vi "FPGA Test.vi"() -> (1 "Resource":string, 2 "ProdName":string)   [LabVIEW 2017]
uses:
  <vilib>/nisyscfg/nisyscfg.lvlib
  <resource>/objmgr/niflexriosae.rc
  <resource>/objmgr/nicriosae.rc
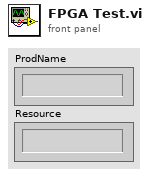
[diagram p1: front panel]
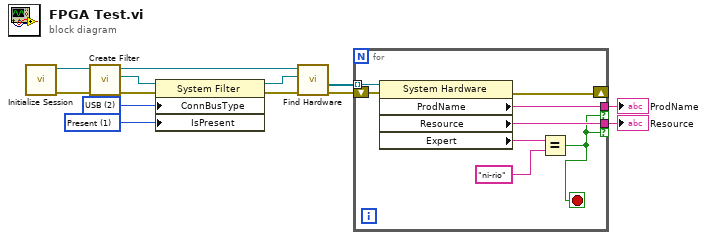
[diagram p0: block diagram]
diagram:
  w6 = 1 items=["Initializing"=-2, "Unknown"=-1, "Not Present"=0, "Present"=1] ("Devices & Chassis:Is Present")
  w7 = u32 2 items=["BuiltIn/System", "PXI/PCI", "USB", "GPIB", "VXI", "Serial", "TCP/IP", "cRIO", "SCXI", "cDAQ", "SwitchBlock", "SCC", "FireWire", "Accessory", "CAN", "SwitchBlock Device"] ("Devices & Chassis:Connects To Bus Type")
  n1 = call <vilib>:"Initialize Session.vi"() -> ("error out"=w5:errorcluster, "Session out"=w9:refnum<k21>)  [unwired: 10 in]
  n2 = call <vilib>:"Create Filter.vi"("error in (no error)"=w5, "Session in"=w9) -> ("error out"=w13:errorcluster, "Filter out"=w12:refnum<k20>, "Session out"=w8:refnum<k21>)  [unwired: 7 in]
  n3 = property class="System Filter"(reference=w12, error in=w13, "ConnBusType"=w7, "IsPresent"=w6) -> (reference out=w11:refnum<k20>, error out=w4:errorcluster)
  n4 = call <vilib>:"Find Hardware.vi"("error in (no error)"=w4, "Filter in"=w11, "Session in"=w8) -> ("error out"=w3:errorcluster, "Resources out"=w10:refnum<k20>[])  [unwired: 5 in, 2 out]
  n5 = for {
    tunnel: w10 -> [w21] mode=indexing
    tunnel: [w20] -> w2 if=w14
    shift-right: [w17] -> _
    shift-left: w3 -> [w18]
    tunnel: [w15] -> w1 if=w14
    stop <- w14 stop-if-true
    n6 = property class="System Hardware"(reference=w21, error in=w18) -> (error out=w17:errorcluster, "ProdName"=w20:string, "Resource"=w15:string, "Expert"=w16:string)  [unwired: 1 out]
    n7 = Equal?(x=w16, y="ni-rio") -> (x = y?=w14:bool)
  }
  "ProdName" <- w2
  "Resource" <- w1
